vi "Bounding Box.vi"(1 "Rects":T1(array[cluster])) -> (0 "Bounding Rect":T2)   [LabVIEW 2011]
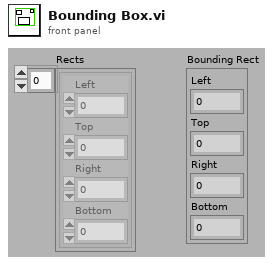
[diagram p1: front panel]
types:
  T1 = cluster{"Left":dbl, "Top":dbl, "Right":dbl, "Bottom":dbl}[]
  T2 = cluster{"Left":dbl, "Top":dbl, "Right":dbl, "Bottom":dbl}
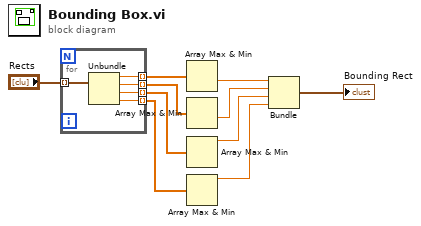
[diagram p0: block diagram]
diagram:
  n1 = for {
    tunnel: "Rects" -> [w15] mode=indexing
    tunnel: [w14] -> w9 mode=indexing
    tunnel: [w13] -> w7 mode=indexing
    tunnel: [w12] -> w6 mode=indexing
    tunnel: [w11] -> w5 mode=indexing
    n2 = Unbundle(w15) -> ("Left"=w14:dbl, "Top"=w13:dbl, "Right"=w12:dbl, "Bottom"=w11:dbl)
  }
  n3 = Array Max & Min(array=w9) -> (min value=w8:dbl)  [unwired: 3 out]
  n4 = Array Max & Min(array=w7) -> (min value=w4:dbl)  [unwired: 3 out]
  n5 = Array Max & Min(array=w6) -> (max value=w3:dbl)  [unwired: 3 out]
  n6 = Array Max & Min(array=w5) -> (max value=w2:dbl)  [unwired: 3 out]
  n7 = Bundle(w8, w4, w3, w2) -> (→"Bounding Rect":cluster{dbl, dbl, dbl, dbl})  [unwired: 1 out]
